vi "Finish.vi"() -> ()   [LabVIEW 2018]
doc: "This VI is called just before exiting. It is expected to close I/O refnum, save collected data, etc."
uses:
  TypeDefs/typedef_enum_Begin.ctl
panel:
  in  "error in":errorcluster
  out "error out":errorcluster
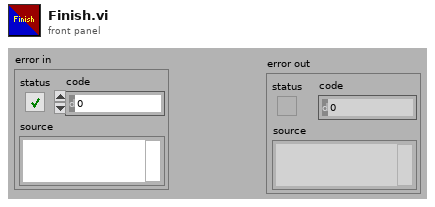
[diagram p1: front panel]
types:
  T1 = typedef "typedef_enum_Begin.ctl" = enum16{"Wrist", "LineFollow", "Gyro", "Climb", "Intake", "Arm", "Drive", "Joysticks"}
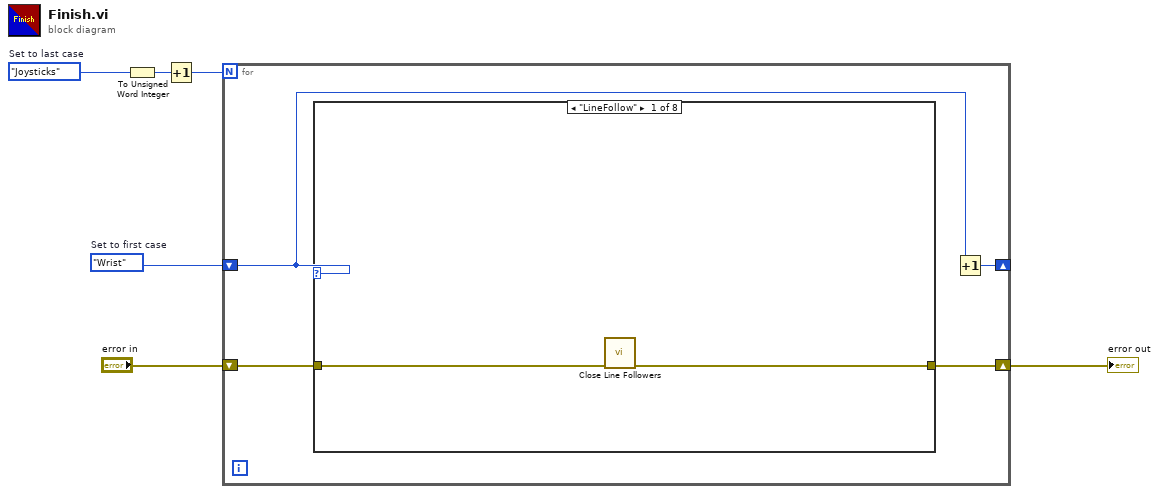
[diagram p0: block diagram]
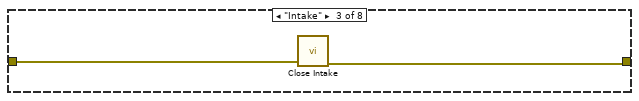
[diagram p3: hidden frame]
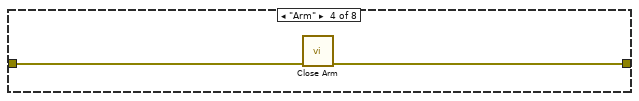
[diagram p4: hidden frame]
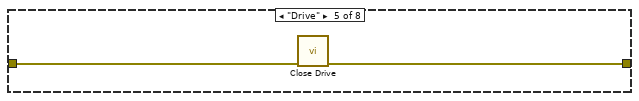
[diagram p5: hidden frame]
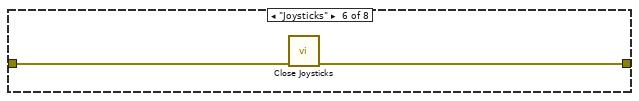
[diagram p6: hidden frame]
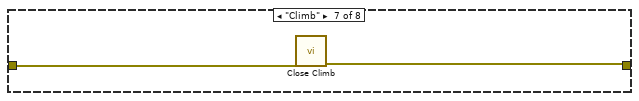
[diagram p7: hidden frame]
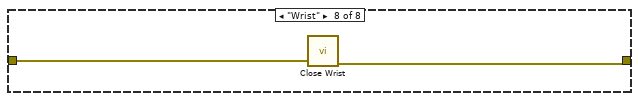
[diagram p8: hidden frame]
diagram:
  w1 = typedef_enum_Begin."Joysticks"  # Set to last case
  w4 = typedef_enum_Begin."Wrist"  # Set to first case
  n1 = To Unsigned Word Integer(number=w1) -> (unsigned 16bit integer=w6:u16)
  n2 = Increment(x=w6) -> (x+1=w5:u16)
  n3 = for {
    N: w5 -> [_]
    shift-right: [w10] -> _
    shift-left: w4 -> [w9]
    shift-right: [w7] -> w2
    shift-left: "error in" -> [w8]
    n4 = case shown="\"LineFollow\"" w9 {
      tunnel: w8 -> [w11 w13 w15 w17 w19 w21 w23 w25]
      tunnel: [w12 w13 w14 w16 w18 w20 w22 w24] -> w7
      frame "LineFollow" {
        n5 = call "Close Line Followers.vi"("error in"=w11) -> ("error out"=w12:errorcluster)  [unwired: 10 in]
      }
      frame "Gyro" {
        # "Don't need to close (no pidgeon IMU close block)"
      }
      frame "Intake" {
        n6 = call "Close Intake.vi"("error in (no error)"=w15) -> ("error out"=w14:errorcluster)  [unwired: 10 in]
      }
      frame "Arm" {
        n7 = call "Close Arm.vi"("error in (no error)"=w17) -> ("error out"=w16:errorcluster)  [unwired: 10 in]
      }
      frame "Drive" {
        n8 = call "Close Drive.vi"("error in"=w19) -> ("error out"=w18:errorcluster)  [unwired: 10 in]
      }
      frame "Joysticks" {
        n9 = call "Close Joysticks.vi"("error in"=w21) -> ("error out"=w20:errorcluster)  [unwired: 10 in]
      }
      frame "Climb" {
        n10 = call "Close Climb.vi"("error in (no error)"=w23) -> ("error out"=w22:errorcluster)  [unwired: 10 in]
      }
      frame "Wrist" {
        n11 = call "Close Wrist.vi"("error in (no error)"=w25) -> ("error out"=w24:errorcluster)  [unwired: 10 in]
      }
    }
    n12 = Increment(x=w9) -> (x+1=w10:T1)
  }
  "error out" <- w2
